vi "VerifyArrayString.vi"(3 "Generated Array":string[](array[string]), 4 "Source Array":string[](array[string]), 5 "String To Append":string) -> (1 "Are All Strings The Expected Strings?":bool)   [LabVIEW 2013]
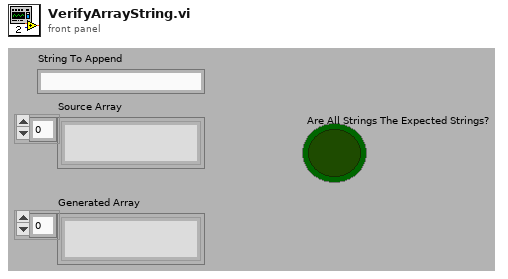
[diagram p1: front panel]
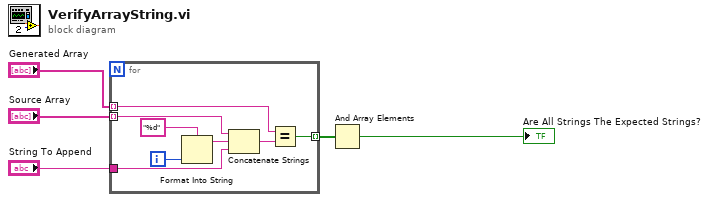
[diagram p0: block diagram]
diagram:
  n1 = for {
    tunnel: "Source Array" -> [w13] mode=indexing
    tunnel: "String To Append" -> [w9]
    tunnel: "Generated Array" -> [w12] mode=indexing
    tunnel: [w10] -> w2 mode=indexing
    i -> [w8]
    n2 = Format Into String(format string="%d", w8) -> (resulting string=w7:string)  [unwired: 2 in, 1 out]
    n3 = Concatenate Strings(w13, w7, w9) -> (w11:string)
    n4 = Equal?(x=w12, y=w11) -> (x = y?=w10:bool)
  }
  n5 = And Array Elements(Boolean array=w2) -> (logical AND=→"Are All Strings The Expected Strings?":bool)
